vi "compare.arrays.vi"(10 "Actual":u64[](array[numeric])=[4702127773838221344, 0] format="%.0x", 11 "Expected":u64[](array[numeric])=[4702127773838221344, 0] format="%.0x") -> (1 "Actual.Out":u64[](array[numeric])=[4702127773838221344, 0] format="%.0x", 2 "Element.Matches":bool[](array[boolean]), 3 "Full.Match":bool)   [LabVIEW 2020]
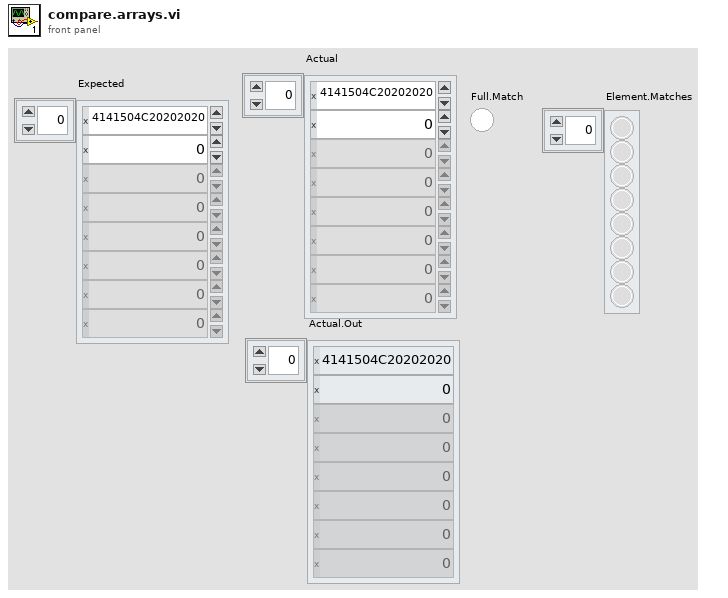
[diagram p1: front panel]
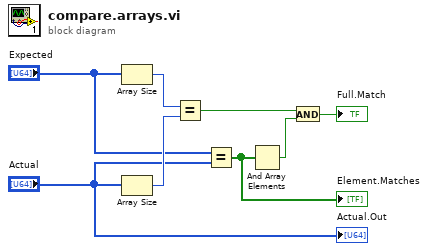
[diagram p0: block diagram]
diagram:
  n1 = Array Size(array="Expected") -> (size(s)=w7:i32)
  n2 = Array Size(array="Actual") -> (size(s)=w6:i32)
  n3 = Equal?(x=w7, y=w6) -> (x = y?=w5:bool)
  n4 = Equal?(x="Expected", y="Actual") -> (x = y?=w8:bool[])
  "Element.Matches" <- w8
  n5 = And Array Elements(Boolean array=w8) -> (logical AND=w4:bool)
  n6 = And(x=w5, y=w4) -> (x .and. y?=→"Full.Match":bool)
  "Actual.Out" <- "Actual"
